vi "Export Origin - LDLTS.vi"(8 "Error In":errorcluster, 9 "Workspace":path, 10 "Session properties":T4, 11 "LDLTS measurement":T1={"Name"="", "Comment"="", "Time"=timestamp(0 s since 1904-01-01), "Folder"=path "", "LDLTS properties"={"T"=0.0, "Test signal"=0.0, "Test frequency"=0.0, "Bandwidth"=0.0, "Averaging"=0.0, "Vbias"=0.0, "Vpulse"=0.0, "pulse length"=0.0, "Pulse 2"=FALSE, "Vpulse 2"=0.0, "pulse length 2"=0.0, "I range"=-2.0, "V range"=10.0, "Sampling rate"=0.0, "Acq. delay"=0.0, "Sampling time"=0.0}, "GUID"=""} {"LDLTS properties"."V range" items=["10mV"=0.01, "100mV"=0.1, "1V"=1.0, "10V"=10.0]; "LDLTS properties"."I range" items=["100nA"=-7.0, "1µA"=-6.0, "10µA"=-5.0, "100µA"=-4.0, "1mA"=-3.0, "10mA"=-2.0]}) -> (0 "Error Out":errorcluster)   [LabVIEW 2019]
doc: "Handles export of a LDLTS measurement to an Origin project, displays a GUI window"
uses:
  Type defs/Session properties Type Def.ctl
  Type defs/LDLTS measurement Type Def.ctl
  Type defs/LDLTS properties Type Def.ctl
  <vilib>/Utility/sysdir.llb/System Directory Type.ctl
panel:
  in  "Comment":T3(array[ring])=[enum."Temperature"] caption="Parameters to be placed in comments"
  in  "Save and exit after export":bool
  in  "Export to current Origin instance":bool
  out "String":string
  in  "Path":path caption="Origin project"
  in  "Export":bool
  in  "Cancel":bool
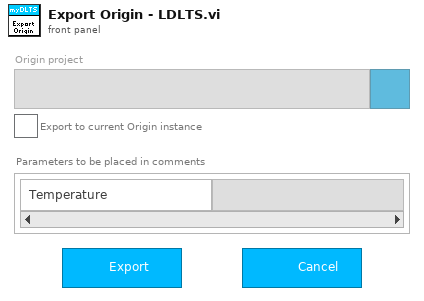
[diagram p1: front panel]
types:
  T1 = typedef "LDLTS measurement Type Def.ctl" = cluster{"Name":string, "Comment":string, "Time":timestamp, "Folder":path, "LDLTS properties":T2, "GUID":string}
  T2 = typedef "LDLTS properties Type Def.ctl" = cluster{"T":dbl[unit], "Test signal":dbl[unit], "Test frequency":dbl[unit], "Bandwidth":dbl[unit], "Averaging":dbl, "Vbias":dbl[unit], "Vpulse":dbl[unit], "pulse length":dbl[unit], "Pulse 2":bool, "Vpulse 2":dbl[unit], "pulse length 2":dbl[unit], "I range":dbl, "V range":dbl[unit], "Sampling rate":dbl[unit], "Acq. delay":dbl[unit], "Sampling time":dbl[unit]}
  T3 = enum16{"", "Temperature", "Test signal", "Test frequency", "Bandwidth", "Averaging", "Bias voltage", "Pulse 1 voltage", "Pulse 1 length", "Pulse 2 voltage", "Pulse 2 length", "Current range", "Voltage range", "Sampling rate", "Acquisition delay"}[]
  T4 = typedef "Session properties Type Def.ctl" = cluster{"Session name":string, "Comment":string, "User":string, "Software version":dbl, "Created":timestamp, "Modified":timestamp, "Binary":bool, "GUID":string}
  T5 = enum32{"existing file", "new file", "new or existing file", "existing dir", "new dir", "new or existing dir", "existing file (use LLBs)", "new file (use LLBs)", "new or existing file (use LLBs)", "new or existing file or directory (use LLBs)", "existing dir (use LLBs)", "new dir (use LLBs)", "new or existing dir (use LLBs)", "existing file or dir", "new file or dir", "new or existing file or dir", "existing file or dir (use LLBs)", "new file or dir (use LLBs)"}
  T6 = typedef "System Directory Type.ctl" = i32
  T7 = enum8{"Enabled", "Disabled", "Disabled and Grayed Out"}
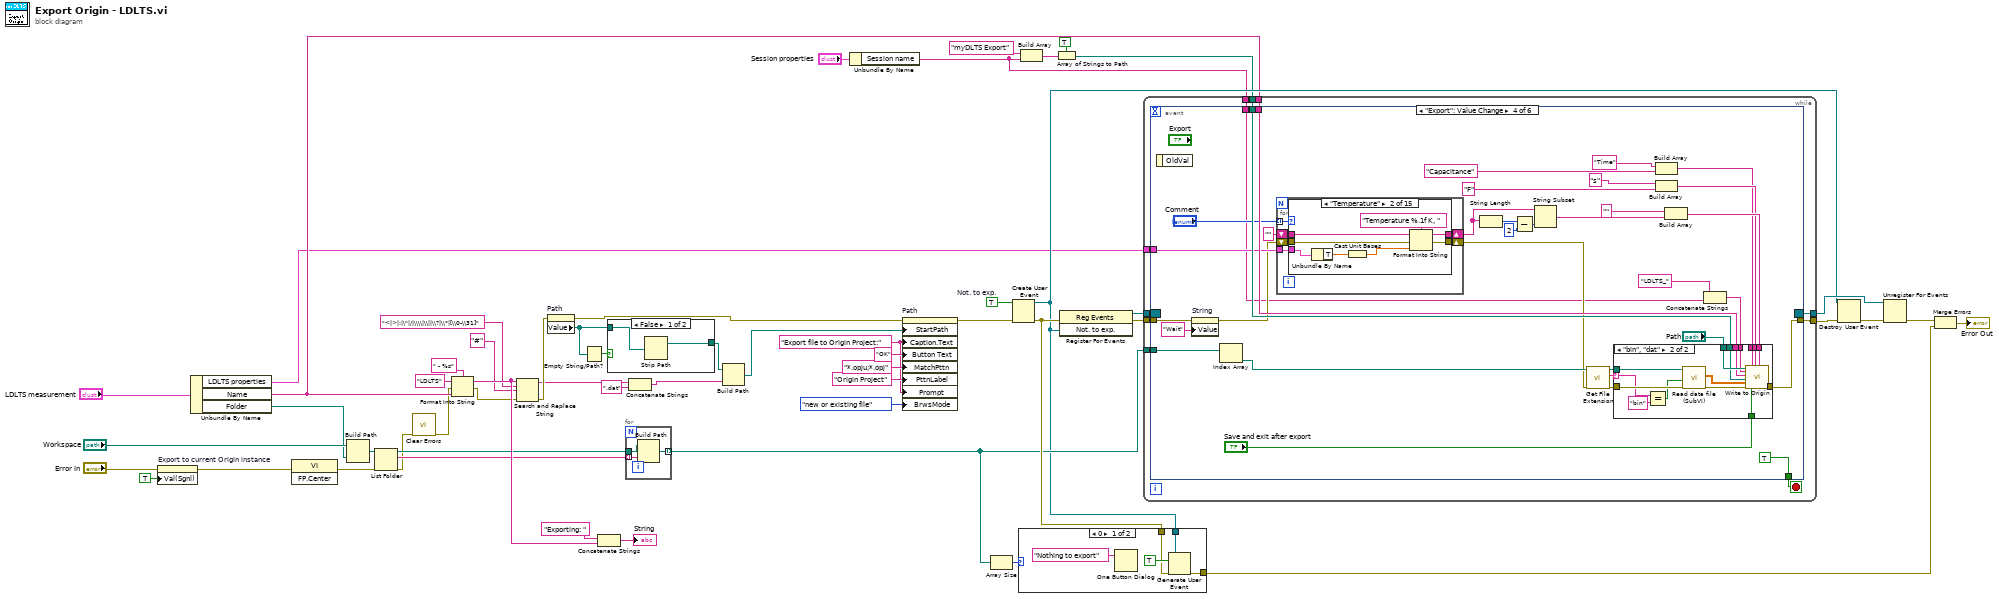
[diagram p0: block diagram]
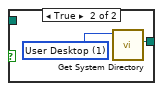
[diagram p2: hidden frame]
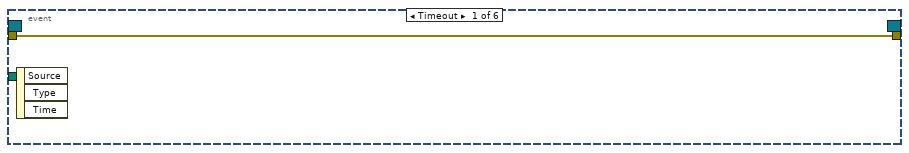
[diagram p4: hidden frame]
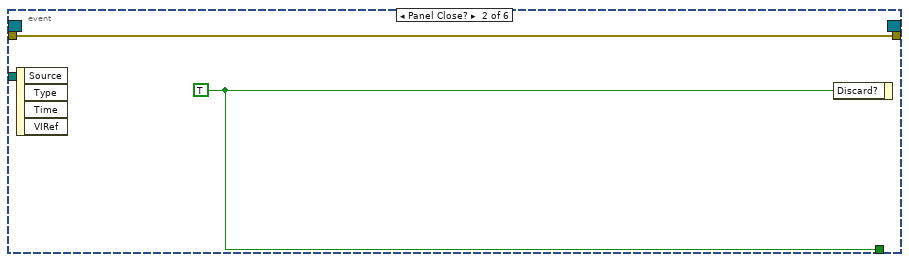
[diagram p5: hidden frame]
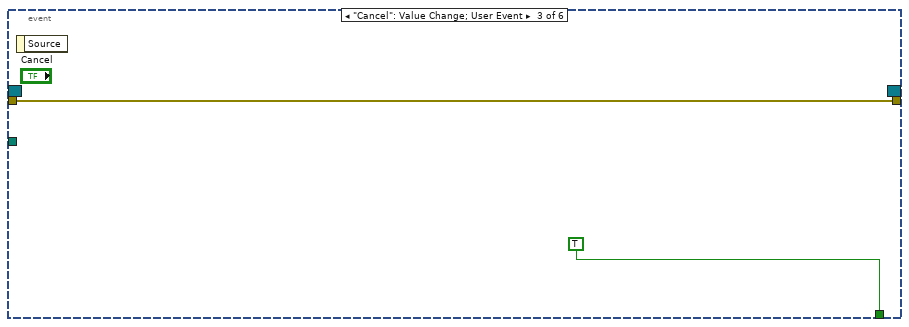
[diagram p6: hidden frame]
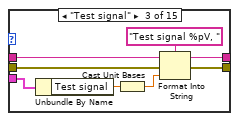
[diagram p8: hidden frame]
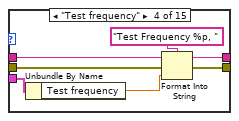
[diagram p9: hidden frame]
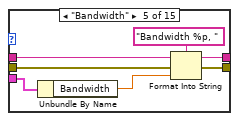
[diagram p10: hidden frame]
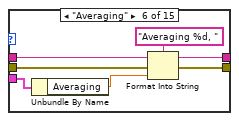
[diagram p11: hidden frame]
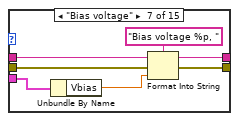
[diagram p12: hidden frame]
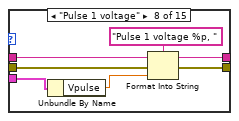
[diagram p13: hidden frame]
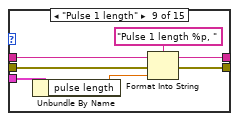
[diagram p14: hidden frame]
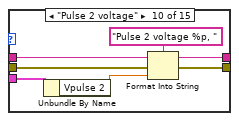
[diagram p15: hidden frame]
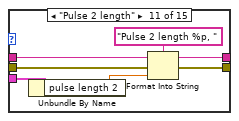
[diagram p16: hidden frame]
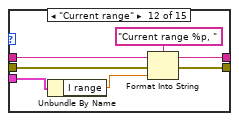
[diagram p17: hidden frame]
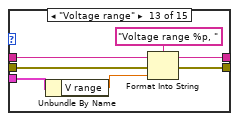
[diagram p18: hidden frame]
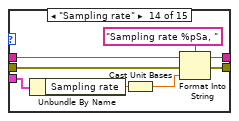
[diagram p19: hidden frame]
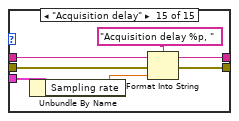
[diagram p20: hidden frame]
diagram:
  w27 = "Export file to Origin Project:"
  w54 = TRUE  # Not. to exp.
  n1 = property on="Export to current Origin instance" class="Bool (strict)"(error in="Error In", "Val(Sgnl)"=TRUE ("Value (Signaling)")) -> (error out=w6:errorcluster)  [unwired: 1 in, 1 out]
  n2 = Unbundle By Name("LDLTS measurement") -> ("LDLTS properties"=w4:T2, "Name"=w14:string, "Folder"=w32:path)
  n3 = invoke class="VI" method="FP.Center"(error in=w6) -> (error out=w16:errorcluster)  [unwired: 2 in, 2 out]
  n4 = Build Path(base path="Workspace", name or relative path=w32) -> (appended path=w25:path)
  n5 = List Folder(path=w25, error in=w16) -> (path out=w24:path, filenames=w31:string[], error out=w20:errorcluster)  [unwired: 2 in, 1 out]
  n6 = call <vilib>:"Clear Errors.vi"("error in (no error)"=w20) -> ("error out"=w1:errorcluster)  [unwired: 5 in, 1 out]
  n7 = Format Into String(format string=" - %s", initial string="LDLTS", error in=w1, w14) -> (resulting string=w43:string, error out=w19:errorcluster)
  n8 = Search and Replace String(input string=w43, search string="<|>|:|\"|/|\\\\|\\||\\?|\\*|[\\0-\\31]", replace string="#" ("replace string (\"\")"), error in=w19) -> (result string=w18:string, error out=w21:errorcluster)  [unwired: 4 in, 2 out]
  n9 = property on="Path" class="Path"(error in=w21) -> (error out=w33:errorcluster, "Value"=w39:path)  [unwired: 1 in, 1 out]
  n10 = Empty String/Path?(string/path=w39) -> (empty?=w40:bool)
  n11 = Concatenate Strings("Exporting: " ("string"), w43) -> (→"String":string)
  n12 = case shown="False" w40 {
    tunnel: w39 -> [w58 _]
    tunnel: [w57 w59] -> w35
    frame False {
      n13 = Strip Path(path=w58) -> (stripped path=w57:path)  [unwired: 1 out]
    }
    frame True {
      w60 = T6 1 items=["User Home"=0, "User Desktop"=1, "User Documents"=2, "User Application Data"=3, "User Preferences"=4, "User Temporary"=5, "Public Documents"=6, "Public Application Data"=7, "Public Preferences"=8, "Public Cache"=13, "System Core Libraries"=9, "System Installed Libraries"=10, "Application Files"=11, "Boot Volume Root"=12] ("system directory type")
      n14 = call <vilib>:"Get System Directory.vi"("system directory type"=w60) -> ("system directory"=w59:path)  [unwired: 10 in]
    }
  }
  n15 = for {
    tunnel: w24 -> [w63]
    tunnel: [w62] -> w49 mode=indexing
    tunnel: w31 -> [w61] mode=indexing
    n16 = Build Path(base path=w63, name or relative path=w61) -> (appended path=w62:path)
  }
  n17 = Concatenate Strings(w18, ".dat" ("string")) -> (w22:string)
  n18 = Build Path(base path=w35, name or relative path=w22) -> (appended path=w34:path)
  n19 = Unbundle By Name("Session properties") -> ("Session name"=w2:string)
  n20 = property on="Path" class="Path"(error in=w33, "StartPath"=w34, "Caption.Text"=w27, "Button Text"="OK", "MatchPttn"="*.opju;*.opj", "PttnLabel"="Origin Project", "Prompt"=w27, "BrwsMode"=T5."new or existing file" ("Browse Options:Selection Mode")) -> (error out=w51:errorcluster)  [unwired: 1 in, 1 out]
  n21 = Array Size(array=w49) -> (size(s)=w55:i32)
  n22 = Create User Event(user event datatype=w54, error in=w51) -> (user event=w15:refnum<user-event>, error out=w50:errorcluster)
  n23 = case shown="0" w55 {
    tunnel: w15 -> [w67 _]
    tunnel: w50 -> [w65 w69]
    tunnel: [w64 w69] -> w44
    frame 0 {
      n24 = One Button Dialog(message="Nothing to export") -> ()  [unwired: 1 in, 1 out]
      n25 = Generate User Event(user event=w67, event data cluster=TRUE ("event data"), error in=w65) -> (error out=w64:errorcluster)  [unwired: 1 in, 1 out]
    }
    frame Default {
    }
  }
  n26 = Build Array("myDLTS Export" ("element"), w2) -> (w10:string[])
  n27 = Array of Strings to Path(0:w10, 1:TRUE ("relative")) -> (2:w9:path)
  n28 = register-events(error in=w50, w15) -> (reference out=w52:refnum<event-registration>, error out=w53:errorcluster)  [unwired: 1 in]
  n29 = while {
    tunnel: w53 -> [w79]
    tunnel: w49 -> [w77]
    tunnel: w52 -> [w76]
    tunnel: [w75] -> w47
    tunnel: w14 -> [w74]
    tunnel: w9 -> [w73]
    tunnel: [w72] -> w8
    tunnel: w4 -> [w71]
    tunnel: w2 -> [w70]
    stop <- w78 stop-if-true
    n30 = event shown="[3] \"Export\": Value Change" {
      selector: w76 -> [_ _ _ _ _ _]
      dyn-events: [_ _ _ _ _ _] -> w75
      timeout: _ -> [_ _ _ _ _ _]
      tunnel: w79 -> [w80 w81 w83 w113 w252 w259]
      tunnel: [w80 w81 w83 w116 w245 w254] -> w72
      tunnel: [_ w82 TRUE ("Discard?") TRUE _ _] -> w78
      tunnel: w77 -> [_ _ _ w118 _ _]
      tunnel: w74 -> [_ _ _ w111 _ _]
      tunnel: w73 -> [_ _ _ w110 _ _]
      tunnel: w71 -> [_ _ _ w95 _ _]
      tunnel: w70 -> [_ _ _ w85 _ _]
      event Timeout {
        n31 = event-data() -> ()  [unwired: 1 in, 3 out]
      }
      event Panel Close? {
        w82 = TRUE ("Discard?")
        n32 = event-data() -> ()  [unwired: 1 in, 4 out]
        n33 = event-data("Discard?"=w82) -> ()  [unwired: 1 in, 1 out]
      }
      event "Cancel": Value Change; User Event {
        n34 = event-data() -> ()  [unwired: 1 in, 1 out]
      }
      event "Export": Value Change {
        n35 = event-data() -> ()  [unwired: 1 in, 1 out]
        n36 = property on="String" class="Str"(error in=w113, "Value"="Wait" ("String")) -> (error out=w94:errorcluster)  [unwired: 1 in, 1 out]
        n37 = Index Array(array=w118) -> (element=w106:path)  [unwired: 1 in]
        n38 = for {
          tunnel: "Comment" -> [w124] mode=indexing
          tunnel: w95 -> [w123]
          shift-right: [w122] -> w93
          shift-left: w94 -> [w121]
          shift-right: [w120] -> w91
          shift-left: "" -> [w119]
          n39 = case shown="\"Temperature\"" w124 {
            tunnel: w123 -> [_ w130 w136 w143 w150 w157 w164 w171 w178 w185 w192 w199 w206 w214 w221]
            tunnel: [w125 w134 w140 w145 w154 w161 w168 w175 w182 w189 w196 w203 w210 w218 w225] -> w122
            tunnel: w121 -> [w125 w132 w138 w147 w152 w159 w165 w172 w179 w186 w193 w200 w207 w215 w222]
            tunnel: [w126 w133 w139 w144 w153 w160 w167 w174 w181 w188 w195 w202 w209 w217 w224] -> w120
            tunnel: w119 -> [w126 w131 w137 w146 w151 w158 w166 w173 w180 w187 w194 w201 w208 w216 w223]
            frame "", Default {
            }
            frame "Temperature" {
              n40 = Unbundle By Name(w130) -> ("T"=w129:dbl[unit])
              n41 = Cast Unit Bases(0:w129) -> (2:w127:dbl)  [unwired: 1 in]
              n42 = Format Into String(format string="Temperature %.1f K, ", initial string=w131, error in=w132, w127) -> (resulting string=w133:string, error out=w134:errorcluster)
            }
            frame "Test signal" {
              n43 = Unbundle By Name(w136) -> ("Test signal"=w141:dbl[unit])
              n44 = Cast Unit Bases(0:w141) -> (2:w135:dbl)  [unwired: 1 in]
              n45 = Format Into String(format string="Test signal %pV, ", initial string=w137, error in=w138, w135) -> (resulting string=w139:string, error out=w140:errorcluster)
            }
            frame "Test frequency" {
              n46 = Unbundle By Name(w143) -> ("Test frequency"=w148:dbl[unit])
              n47 = Format Into String(format string="Test Frequency %p, ", initial string=w146, error in=w147, w148) -> (resulting string=w144:string, error out=w145:errorcluster)
            }
            frame "Bandwidth" {
              n48 = Unbundle By Name(w150) -> ("Bandwidth"=w155:dbl[unit])
              n49 = Format Into String(format string="Bandwidth %p, ", initial string=w151, error in=w152, w155) -> (resulting string=w153:string, error out=w154:errorcluster)
            }
            frame "Averaging" {
              n50 = Unbundle By Name(w157) -> ("Averaging"=w162:dbl)
              n51 = Format Into String(format string="Averaging %d, ", initial string=w158, error in=w159, w162) -> (resulting string=w160:string, error out=w161:errorcluster)
            }
            frame "Bias voltage" {
              n52 = Unbundle By Name(w164) -> ("Vbias"=w169:dbl[unit])
              n53 = Format Into String(format string="Bias voltage %p, ", initial string=w166, error in=w165, w169) -> (resulting string=w167:string, error out=w168:errorcluster)
            }
            frame "Pulse 1 voltage" {
              n54 = Unbundle By Name(w171) -> ("Vpulse"=w176:dbl[unit])
              n55 = Format Into String(format string="Pulse 1 voltage %p, ", initial string=w173, error in=w172, w176) -> (resulting string=w174:string, error out=w175:errorcluster)
            }
            frame "Pulse 1 length" {
              n56 = Unbundle By Name(w178) -> ("pulse length"=w183:dbl[unit])
              n57 = Format Into String(format string="Pulse 1 length %p, ", initial string=w180, error in=w179, w183) -> (resulting string=w181:string, error out=w182:errorcluster)
            }
            frame "Pulse 2 voltage" {
              n58 = Unbundle By Name(w185) -> ("Vpulse 2"=w190:dbl[unit])
              n59 = Format Into String(format string="Pulse 2 voltage %p, ", initial string=w187, error in=w186, w190) -> (resulting string=w188:string, error out=w189:errorcluster)
            }
            frame "Pulse 2 length" {
              n60 = Unbundle By Name(w192) -> ("pulse length 2"=w197:dbl[unit])
              n61 = Format Into String(format string="Pulse 2 length %p, ", initial string=w194, error in=w193, w197) -> (resulting string=w195:string, error out=w196:errorcluster)
            }
            frame "Current range" {
              n62 = Unbundle By Name(w199) -> ("I range"=w204:dbl)
              n63 = Format Into String(format string="Current range %p, ", initial string=w201, error in=w200, w204) -> (resulting string=w202:string, error out=w203:errorcluster)
            }
            frame "Voltage range" {
              n64 = Unbundle By Name(w206) -> ("V range"=w211:dbl[unit])
              n65 = Format Into String(format string="Voltage range %p, ", initial string=w208, error in=w207, w211) -> (resulting string=w209:string, error out=w210:errorcluster)
            }
            frame "Sampling rate" {
              n66 = Unbundle By Name(w214) -> ("Sampling rate"=w219:dbl[unit])
              n67 = Cast Unit Bases(0:w219) -> (2:w213:dbl)  [unwired: 1 in]
              n68 = Format Into String(format string="Sampling rate %pSa, ", initial string=w216, error in=w215, w213) -> (resulting string=w217:string, error out=w218:errorcluster)
            }
            frame "Acquisition delay" {
              n69 = Unbundle By Name(w221) -> ("Sampling rate"=w226:dbl[unit])
              n70 = Format Into String(format string="Acquisition delay %p, ", initial string=w223, error in=w222, w226) -> (resulting string=w224:string, error out=w225:errorcluster)
            }
          }
        }
        n71 = String Length(string=w91) -> (length=w90:i32)
        n72 = Subtract(x=w90, y=2) -> (x-y=w89:i32)
        n73 = String Subset(string=w91, length (rest)=w89) -> (substring=w102:string)  [unwired: 1 in]
        n74 = call <vilib>:"Get File Extension.vi"("error in (no error)"=w93, "file"=w106) -> ("error out"=w108:errorcluster, "lowercase file extension"=w107:string, "dup file"=w109:path)  [unwired: 5 in, 2 out]
        n75 = Build Array("Time", "Capacitance") -> (w96:string[])
        n76 = Build Array("s", "F") -> (w97:string[])
        n77 = Build Array("", w102) -> (w98:string[])
        n78 = Concatenate Strings("LDLTS_" ("Book name"), w85) -> (w86:string)
        n79 = case shown="\"bin\", \"dat\"" w107 {
          selector: w107 -> [_ w229]
          tunnel: w109 -> [_ w243]
          tunnel: w108 -> [w228 w242]
          tunnel: "Path" -> [_ w238]
          tunnel: w96 -> [_ w237]
          tunnel: w97 -> [_ w236]
          tunnel: w98 -> [_ w235]
          tunnel: [w228 w234] -> w116
          tunnel: "Save and exit after export" -> [_ w233]
          tunnel: w86 -> [_ w232]
          tunnel: w111 -> [_ w231]
          tunnel: w110 -> [_ w230]
          frame "False", Default {
          }
          frame "bin", "dat" {
            n80 = Equal?(x=w229, y="bin") -> (x = y?=w241:bool)
            n81 = call "Read data file (SubVI).vi"("error in"=w242, "Binary"=w241, "file path in"=w243) -> ("error out"=w239:errorcluster, "2D data"=w240:dbl[][])  [unwired: 6 in, 1 out]
            n82 = call "Write to Origin.vi"("Origin Project Path"=w238, "Book name"=w232, "Sheet name"=w231, "Folder name"=w230, "Data"=w240, "error in (no error)"=w239, "Column name"=w237, "Save and exit"=w233, "Column unit"=w236, "Column comment"=w235) -> ("error out"=w234:errorcluster)  [unwired: 9 in]
          }
        }
      }
      event "Export to current Origin instance": Value Change {
        n83 = event-data() -> ("NewVal"=w247:bool)  [unwired: 1 in]
        n84 = Select(t=T7."Disabled and Grayed Out" ("Disabled"), s=w247, f=T7."Enabled" ("Disabled")) -> (s? t:f=w248:T7)
        n85 = property on="Path" class="Path"(error in=w252, "Val(Sgnl)"=path "" ("Value (Signaling)"), "DisabledEnum"=w248) -> (error out=w251:errorcluster)  [unwired: 1 in, 1 out]
        n86 = Not(x=w247) -> (.not. x?=w246:bool)
        n87 = property on="Save and exit after export" class="Bool (strict)"(error in=w251, "Visible"=w246) -> (error out=w245:errorcluster)  [unwired: 1 in, 1 out]
      }
      event "Path": Value Change {
        n88 = event-data() -> ("NewVal"=w263:path)  [unwired: 1 in]
        n89 = Path Type(1:w263) -> (0:w262:i16)
        n90 = Equal To 0?(x=w262) -> (x = 0?=w260:bool)
        n91 = Or(x=w260, y="Export to current Origin instance") -> (x .or. y?=w258:bool)
        n92 = Select(t=T7."Enabled" ("Disabled"), s=w258, f=T7."Disabled and Grayed Out") -> (s? t:f=w257:T7)
        n93 = property on="Export" class="Bool"(error in=w259, "DisabledEnum"=w257) -> (error out=w254:errorcluster)  [unwired: 1 in, 1 out]
      }
    }
  }
  n94 = Destroy User Event(user event=w15, error in=w8) -> (error out=w48:errorcluster)
  n95 = Unregister For Events(event registration refnum=w47, error in=w48) -> (error out=w46:errorcluster)
  n96 = Merge Errors(w46, w44) -> (→"Error Out":errorcluster)
